vi "DCPower_MeasureRecordConfiguration.vi"(7 "Aperture Time":dbl, 8 "error in (no error)":errorcluster, 9 "Measure Record Length":i32, 10 "Active Channel Numbers String":string, 11 "IVI Refnum in":refnum<k15>) -> (0 "error out":errorcluster, 3 "IVI Refnum out":refnum<k15>)   [LabVIEW 2019]
uses:
  <instrlib>/niDCPower/nidcpower.llb/niDCPower Aperture Time Units.ctl
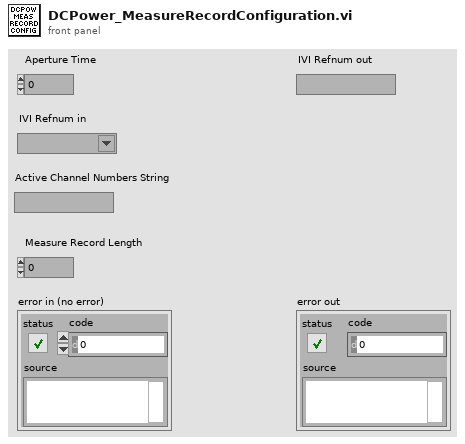
[diagram p1: front panel]
types:
  T1 = typedef "niDCPower Aperture Time Units.ctl" = i32
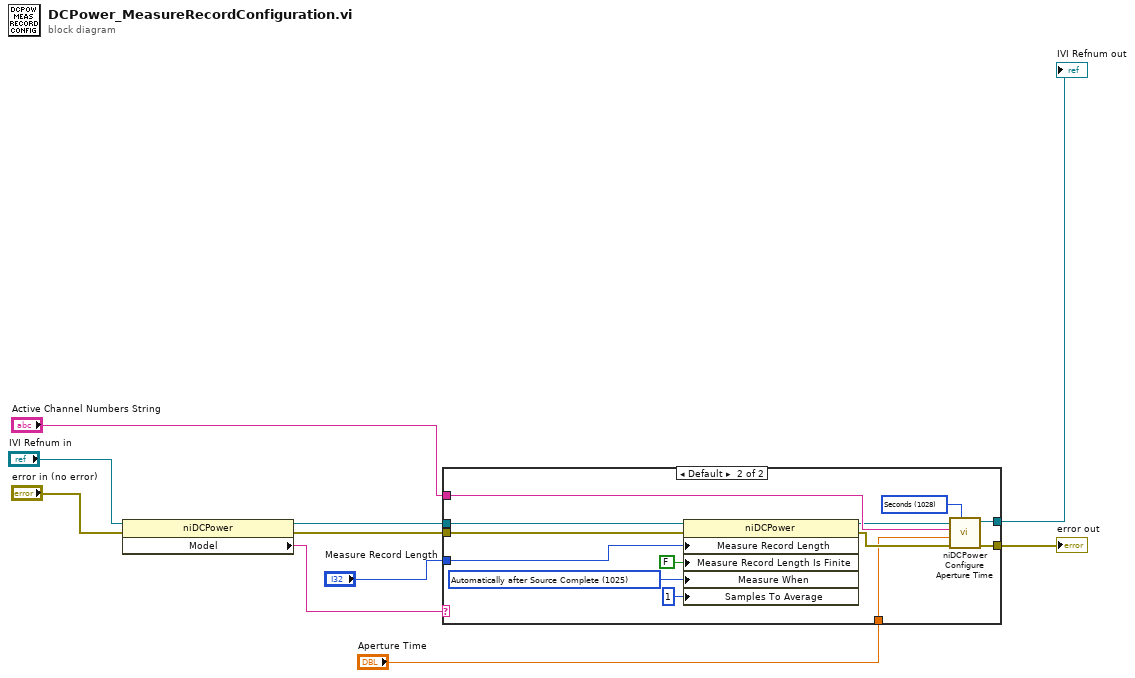
[diagram p0: block diagram]
diagram:
  n1 = property class="niDCPower"(reference="IVI Refnum in", error in="error in (no error)") -> (reference out=w2:refnum<k15>, error out=w3:errorcluster, "Model"=w4:string)
  n2 = case shown="Default" w4 {
    tunnel: [w11 w24] -> w10
    tunnel: [w12 w23] -> w9
    tunnel: "Active Channel Numbers String" -> [_ w22]
    tunnel: w2 -> [w12 w18]
    tunnel: w3 -> [w11 w17]
    tunnel: "Aperture Time" -> [_ w14]
    tunnel: "Measure Record Length" -> [_ w13]
    frame "NI PXI-4110", "NI PXI-4130", "NI PXI-4131A", "NI PXIe-4154" {
    }
    frame Default {
      w20 = 1025 items=["Automatically after Source Complete"=1025, "On Demand"=1026, "On Measure Trigger"=1027] ("Measurement:Advanced:Measure When")
      w25 = T1 1028 items=["Seconds"=1028, "Powerline Cycles"=1029] ("aperture time units")
      n3 = property class="niDCPower"(reference=w18, error in=w17, "Measure Record Length"=w13, "Measure Record Length Is Finite"=FALSE ("Measurement:Measure Record Length Is Finite"), "Measure When"=w20, "Samples To Average"=1 ("Measurement:Samples To Average")) -> (reference out=w16:refnum<k15>, error out=w15:errorcluster)
      n4 = call <instrlib>:"niDCPower Configure Aperture Time.vi"("aperture time units"=w25, "error in (no error)"=w15, "aperture time"=w14, "channel name"=w22, "instrument handle"=w16) -> ("error out"=w24:errorcluster, "instrument handle out"=w23:refnum<k15>)  [unwired: 5 out]
    }
  }
  "error out" <- w10
  "IVI Refnum out" <- w9
